vi "mark.vi"(0 "Image In":T2, 1 "Group":string, 2 "Point":T1 {"Y" format="%.2f"; "X" format="%.2f"}, 3 "String":string="  Start", 4 "Text Color (black)":u32(colorbox)=16860) -> (5 "Image Out":T2)   [LabVIEW 2014]
doc: "在二维图中标记起点或终点"
uses:
  <vilib>/vision/Image Controls.llb/IMAQ Image.ctl
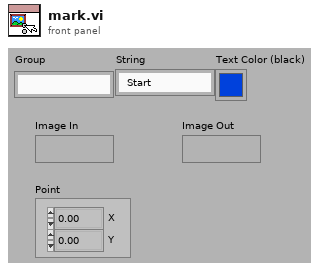
[diagram p1: front panel]
types:
  T1 = typedef "IMAQ Point" = cluster{"X":sgl, "Y":sgl}
  T2 = typedef "IMAQ Image.ctl" = refnum<image>
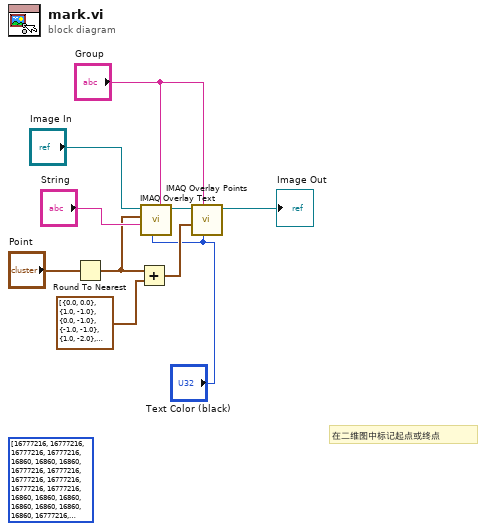
[diagram p0: block diagram]
diagram:
  (unwired) u32[][] [[16777216, 16777216, 16777216, 16777216, 16860, 16860, 16860, 16777216, 16777216, 16777216, 16777216], [16777216, 16777216, 16860, 16860, 16860, 16860, 16860, 16860, 16860, 16777216, 16777216], [16777216, 16860, 16860, 16860, 16860, 16860, 16860, 16860, 16860, 16860, 16777216], [16860, 16860, 16860, 16860, 16777216, 16777216, 16777216, 16860, 16860, 16860, 16860], [16860, 16860, 16860, 16777216, 16777216, 16777216, 16777216, 16777216, 16860, 16860, 16860], [16860, 16860, 16860, 16777216, 16777216, 16777216, 16777216, 16777216, 16860, 16860, 16860], [16777216, 16860, 16860, 16860, 16777216, 16777216, 16777216, 16860, 16860, 16860, 16777216], [16777216, 16777216, 16860, 16860, 16860, 16777216, 16860, 16860, 16860, 16777216, 16777216], [16777216, 16777216, 16777216, 16860, 16860, 16860, 16860, 16860, 16777216, 16777216, 16777216], [16777216, 16777216, 16777216, 16860, 16860, 16860, 16860, 16860, 16777216, 16777216, 16777216], [16777216, 16777216, 16777216, 16777216, 16860, 16860, 16860, 16777216, 16777216, 16777216, 16777216], [16777216, 16777216, 16777216, 16777216, 16860, 16860, 16860, 16777216, 16777216, 16777216, 16777216], [16777216, 16777216, 16777216, 16777216, 16777216, 16860, 16777216, 16777216, 16777216, 16777216, 16777216]] ("Bitmap")
  # "在二维图中标记起点或终点"
  n1 = Round To Nearest(number="Point") -> (nearest integer value=w1:T1)
  n2 = Add(x=w1, y=cluster{sgl, sgl}[] [{0.0, 0.0}, {1.0, -1.0}, {0.0, -1.0}, {-1.0, -1.0}, {1.0, -2.0}, {0.0, -2.0}, {-1.0, -2.0}, {2.0, -3.0}, {1.0, -3.0}, {0.0, -3.0}, {-1.0, -3.0}, {-2.0, -3.0}, {2.0, -4.0}, {1.0, -4.0}, {0.0, -4.0}, {-1.0, -4.0}, {-2.0, -4.0}, {3.0, -5.0}, {2.0, -5.0}, {1.0, -5.0}, {-1.0, -5.0}, {-2.0, -5.0}, {-3.0, -5.0}, {4.0, -6.0}, {3.0, -6.0}, {2.0, -6.0}, {-2.0, -6.0}, {-3.0, -6.0}, {-4.0, -6.0}, {5.0, -7.0}, {4.0, -7.0}, {3.0, -7.0}, {-3.0, -7.0}, {-4.0, -7.0}, {-5.0, -7.0}, {5.0, -8.0}, {4.0, -8.0}, {3.0, -8.0}, {-3.0, -8.0}, {-4.0, -8.0}, {-5.0, -8.0}, {5.0, -9.0}, {4.0, -9.0}, {3.0, -9.0}, {2.0, -9.0}, {-2.0, -9.0}, {-3.0, -9.0}, {-4.0, -9.0}, {-5.0, -9.0}, {4.0, -10.0}, {3.0, -10.0}, {2.0, -10.0}, {1.0, -10.0}, {0.0, -10.0}, {-1.0, -10.0}, {-2.0, -10.0}, {-3.0, -10.0}, {-4.0, -10.0}, {3.0, -11.0}, {2.0, -11.0}, {1.0, -11.0}, {0.0, -11.0}, {-1.0, -11.0}, {-2.0, -11.0}, {-3.0, -11.0}, {1.0, -12.0}, {0.0, -12.0}, {-1.0, -12.0}] ("数组")) -> (x+y=w10:T1[])
  n3 = call "IMAQ Overlay Text"("Group"="Group", "Text Color (black)"="Text Color (black)", "String"="String", "Origin"=w1, "Image"="Image In") -> ("Image Out"=w7:T2)  [unwired: 5 in, 1 out]
  n4 = call "IMAQ Overlay Points"("Color"="Text Color (black)", "Group"="Group", "Array of Points"=w10, "Image"=w7) -> ("Image Out"=→"Image Out":T2)  [unwired: 6 in, 1 out]
